vi "rmx13_rev2 - Copy.vi"() -> ()   [LabVIEW 2012]
uses:
  <vilib>/Utility/inputDevices.llb/closeKeyboard.vi
  <vilib>/Utility/inputDevices.llb/keyboardAcquire.vi
panel:
  in  "Tab Control":enum32{"Front Panel"}(tab)
  out "excavator direction":string="a"
  out "bot direction":string="a"
  out "excavator state":string="a"
  out "hopper state":string="a"
  out "bytes written":i32
  out "tx'd string":string
  out "error out":errorcluster
  in  "Boolean 2":bool
  in  "Boolean":bool
  out "Total Elapsed Time  (HH:MM:SS)":dbl format="%<%H:%M:%S%2u>t"
  out "hup":bool
  out "hdown":bool
  out "xfwd":bool
  out "xback":bool
  out "xdown":bool
  out "xup":bool
  out "right":bool
  out "left":bool
  out "down":bool
  out "up":bool
  # "Excavator State"
  # "Elapsed Time"
  # "Error Control"
  # "Dump Position"
  # "Excavator Direction"
  # "Start/Stop"
  # "Bot Direction"
  # "Hopper State"
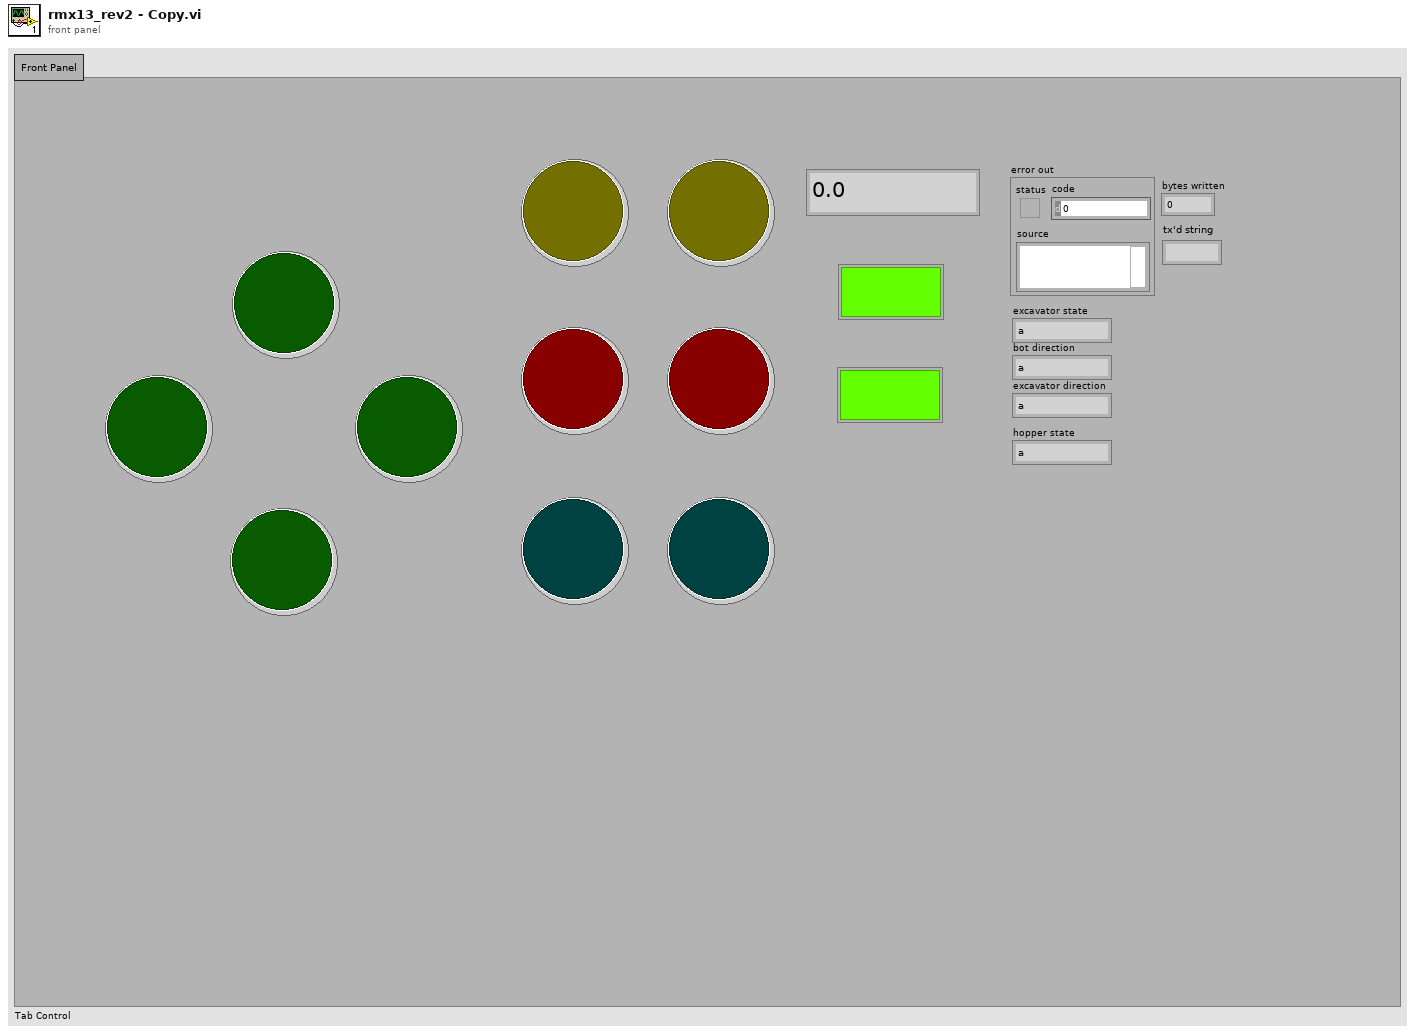
[diagram p1: front panel]
types:
  T1 = enum16{"0", "1", "2", "3", "4", "5", "6", "7", "8", "9", "A", "B", "C", "D", "E", "F", "G", "H", "I", "J", "K", "L", "M", "N", "O", "P", "Q", "R", "S", "T", "U", "V", "W", "X", "Y", "Z", "F1", "F2", "F3", "F4", "F5", "F6", "F7", "F8", "F9", "F10", "F11", "F12", "F13", "F14", "F15", "ADD", "BACK", "BACKSLASH", "CAPITAL", "COMMA", "DECIMAL", "DELETE", "DIVIDE", "DOWN", "END", "EQUALS", "ESCAPE", "GRAVE (`)", "HOME", "INSERT", "LBRACKET", "LCONTROL", "LEFT", "L ALT", "LSHIFT", "LWIN", "MINUS", "MULTIPLY", "NEXT", "NUMLOCK", "NUMPAD_0", "NUMPAD_1", "NUMPAD_2", "NUMPAD_3", "NUMPAD_4", "NUMPAD_5", "NUMPAD_6", "NUMPAD_7", "NUMPAD_8", "NUMPAD_9", "PAUSE", "PERIOD", "PRIOR (PG UP)", "RBRACKET", "RCONTROL", "RETURN", "RIGHT", "R ALT", "RSHIFT", "RWIN", "SCROLL", "SEMICOLON", "SLASH", "SPACE", "SUBTRACT", "TAB", "UP", "ENTER (num pad)", "' (quote)"}[]
  T2 = cluster{"up":bool, "down":bool, "left":bool, "right":bool, "xup":bool, "xdown":bool, "hup":bool, "hdown":bool, "xfwd":bool, "xback":bool}
  T3 = cluster{"bot_dir":string, "x-state":string, "h-state":string, "x-dir":string}
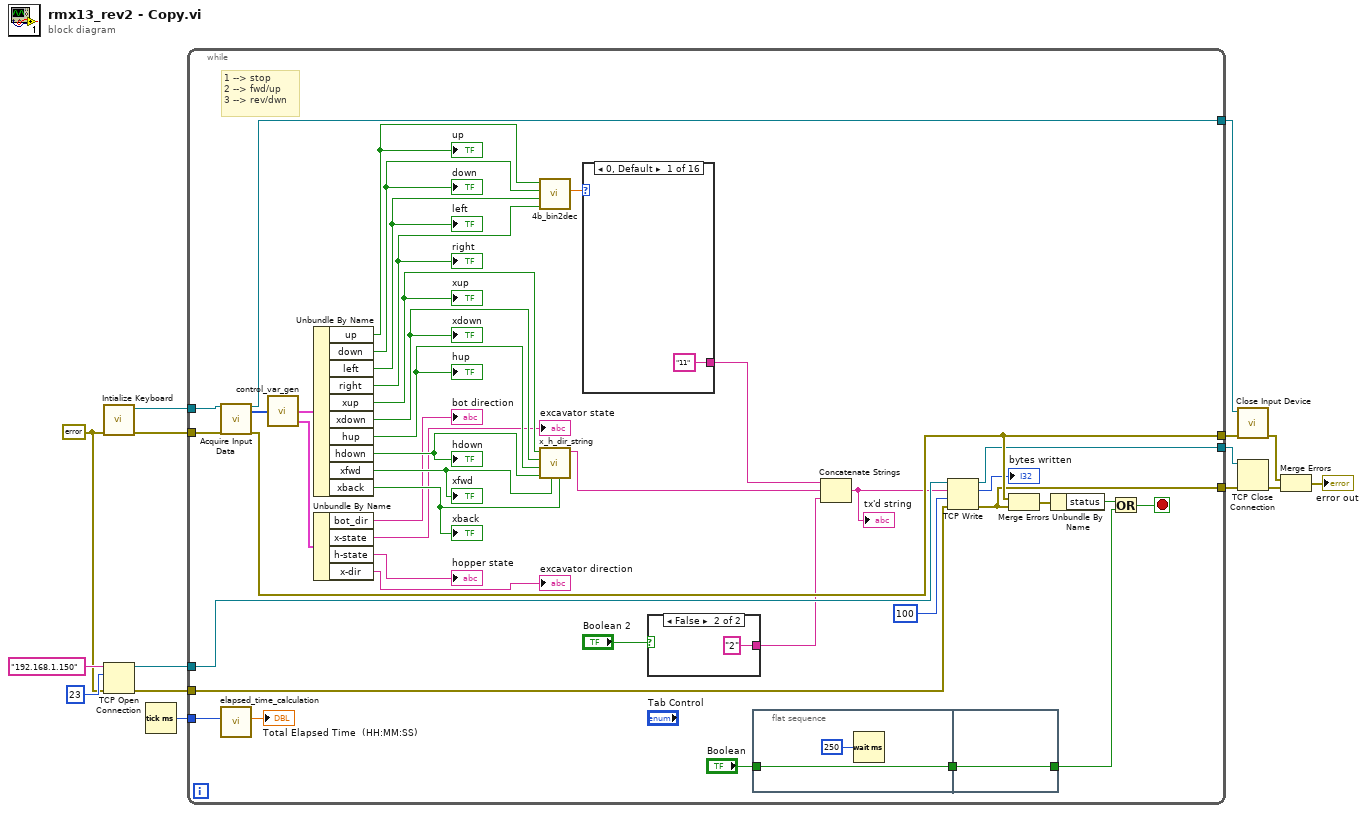
[diagram p0: block diagram]
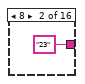
[diagram p2: hidden frame]
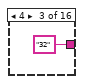
[diagram p3: hidden frame]
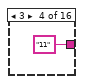
[diagram p4: hidden frame]
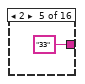
[diagram p5: hidden frame]
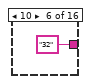
[diagram p6: hidden frame]
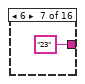
[diagram p7: hidden frame]
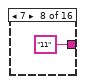
[diagram p8: hidden frame]
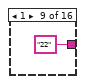
[diagram p9: hidden frame]
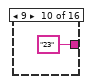
[diagram p10: hidden frame]
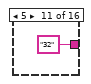
[diagram p11: hidden frame]
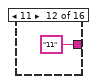
[diagram p12: hidden frame]
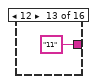
[diagram p13: hidden frame]
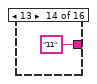
[diagram p14: hidden frame]
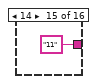
[diagram p15: hidden frame]
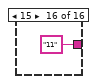
[diagram p16: hidden frame]
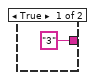
[diagram p17: hidden frame]
diagram:
  w3 = errorcluster {"status"=FALSE, "code"=0, "source"=""} ("error in")
  n1 = call <vilib>:"Intialize Keyboard.vi"("error in (no error)"=w3) -> ("error out"=w14:errorcluster, "device ID"=w15:refnum<k1>)  [unwired: 9 in]
  n2 = TCP Open Connection(address="192.168.1.150", remote port or service name=u16 23, error in (no error)=w3) -> (connection ID=w6:refnum<k5>, error out=w7:errorcluster)  [unwired: 2 in]
  n3 = Tick Count (ms)() -> (millisecond timer value=w11:u32)
  n4 = while {
    tunnel: w15 -> [w56]
    tunnel: w14 -> [w55]
    tunnel: [w52] -> w13
    tunnel: [w45] -> w12
    tunnel: w11 -> [w43]
    tunnel: w7 -> [w30]
    tunnel: w6 -> [w29]
    tunnel: [w27] -> w5
    tunnel: [w24] -> w4
    stop <- w46 stop-if-true
    # "1 --> stop\n2 --> fwd/up\n3 --> rev/dwn"
    n5 = call-poly <vilib>:"Acquire Input Data.vi"("device ID"=w56, "error in (no error)"=w55) -> ("device ID"=w52:refnum<k1>, "keys pressed"=w51:T1, "error out"=w45:errorcluster)  [unwired: 15 in]
    n6 = call "elapsed_time_calculation.vi"("initial time"=w43) -> ("elapsed time"=→"Total Elapsed Time  (HH:MM:SS)":dbl)  [unwired: 10 in]
    n7 = call "control_var_gen.vi"("keys pressed"=w51) -> ("out_panel"=w50:T2, "out_error"=w49:T3)  [unwired: 5 in]
    n8 = Unbundle By Name(w50) -> ("up"=w41:bool, "down"=w40:bool, "left"=w39:bool, "right"=w38:bool, "xup"=w37:bool, "xdown"=w36:bool, "hup"=w35:bool, "hdown"=w34:bool, "xfwd"=w33:bool, "xback"=w32:bool)
    "up" <- w41
    "down" <- w40
    "left" <- w39
    "right" <- w38
    "xup" <- w37
    "xdown" <- w36
    "hup" <- w35
    "hdown" <- w34
    "xfwd" <- w33
    "xback" <- w32
    n9 = Unbundle By Name(w49) -> ("bot_dir"=→"bot direction":string, "x-state"=→"excavator state":string, "h-state"=→"hopper state":string, "x-dir"=→"excavator direction":string)
    n10 = call "4b_bin2dec.vi"("Right"=w38, "Left"=w39, "Down"=w40, "Up"=w41) -> ("Out"=w17:dbl)  [unwired: 7 in]
    n11 = call "x_h_dir_string.vi"("xback"=w32, "xfwd"=w33, "hdown"=w34, "hup"=w35, "xdown"=w36, "xup"=w37) -> ("x_h_dir"=w31:string)  [unwired: 5 in]
    n12 = case shown="0, Default" w17 {
      tunnel: ["11" ("motor_control_sig") "23" ("motor_control_sig") "32" ("motor_control_sig") "11" ("motor_control_sig") "33" ("motor_control_sig") "32" ("motor_control_sig") "23" ("motor_control_sig") "11" ("motor_control_sig") "22" ("motor_control_sig") "23" ("motor_control_sig") "32" ("motor_control_sig") "11" ("motor_control_sig") "11" ("motor_control_sig") "11" ("motor_control_sig") "11" ("motor_control_sig") "11" ("motor_control_sig")] -> w16
      frame 0, Default {
      }
      frame 8 {
      }
      frame 4 {
      }
      frame 3 {
      }
      frame 2 {
      }
      frame 10 {
      }
      frame 6 {
      }
      frame 7 {
      }
      frame 1 {
      }
      frame 9 {
      }
      frame 5 {
      }
      frame 11 {
      }
      frame 12 {
      }
      frame 13 {
      }
      frame 14 {
      }
      frame 15 {
      }
    }
    n13 = case shown="False" "Boolean 2" {
      tunnel: ["3" "2"] -> w25
      frame True {
      }
      frame False {
      }
    }
    n14 = flat-sequence {
      tunnel: "Boolean" -> [w75]
      tunnel: [w75] -> w54
      tunnel: [w77] -> w47
      tunnel: w54 -> [w77]
      frame #0 {
        n15 = Wait (ms)(milliseconds to wait=u32 250) -> ()  [unwired: 1 out]
      }
      frame #1 {
      }
    }
    n16 = Concatenate Strings(w16, w31, w25) -> (w18:string)
    "tx'd string" <- w18
    n17 = TCP Write(connection ID=w29, data in=w18, error in (no error)=w30, 9:100 ("timeout ms (25000)")) -> (connection ID out=w27:refnum<k5>, bytes written=→"bytes written":i32, error out=w24:errorcluster)
    n18 = Merge Errors(w45, w24) -> (w44:errorcluster)
    n19 = Unbundle By Name(w44) -> ("status"=w48:bool)
    n20 = Or(x=w48, y=w47) -> (x .or. y?=w46:bool)
  }
  n21 = call-poly <vilib>:"Close Input Device.vi"("error in (no error)"=w12, "device ID"=w13) -> ("error out"=w10:errorcluster)  [unwired: 8 in]
  n22 = TCP Close Connection(connection ID=w5, error in (no error)=w4) -> (error out=w2:errorcluster)  [unwired: 1 in, 1 out]
  n23 = Merge Errors(w10, w2) -> (→"error out":errorcluster)
